vi "ReadIOIni.vi"(11 "IOPathIn":path) -> (3 "DIO":cluster{"DI=1":i32, "Name":string[]}[](array[cluster]))   [LabVIEW 2019]
uses:
  <vilib>/Utility/config.llb/Read Key (String).vi
  <vilib>/Utility/config.llb/NI_LVConfig.lvlib
panel:
  out "Numeric":i32
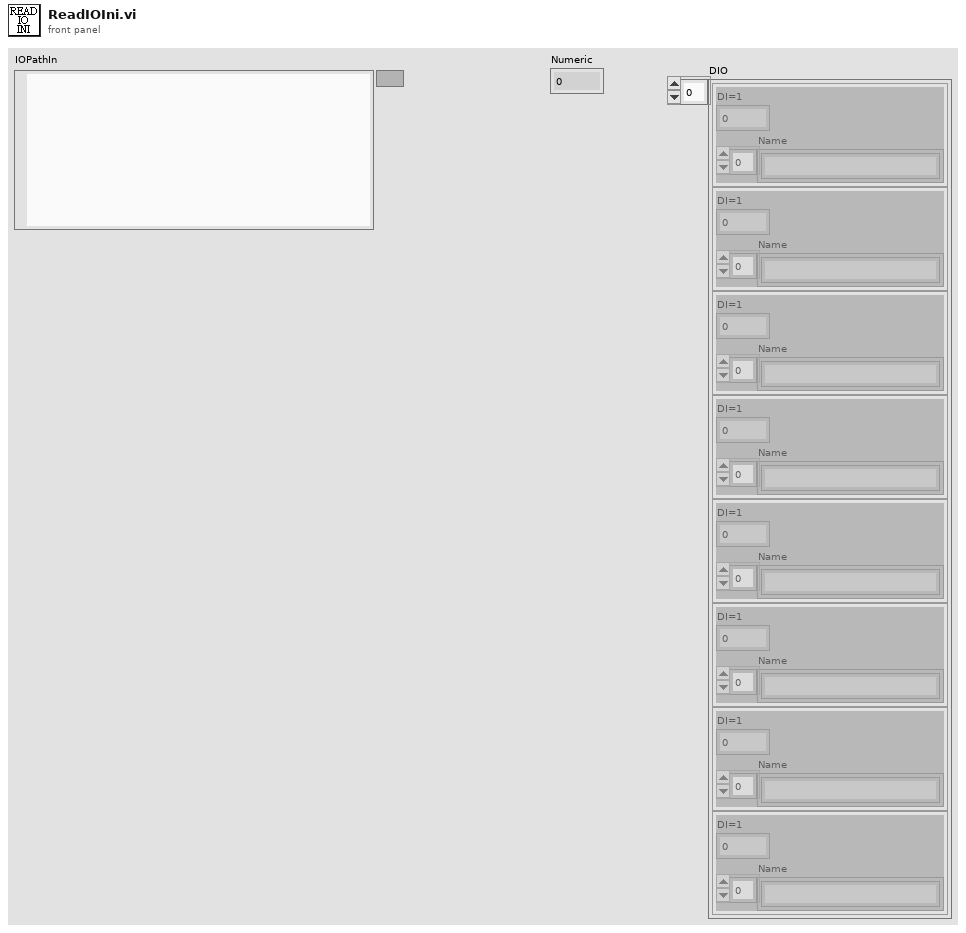
[diagram p1: front panel]
types:
  T1 = typedef "NI_LVConfig.lvlib/Config Data RefNum.ctl" = refnum<k1>
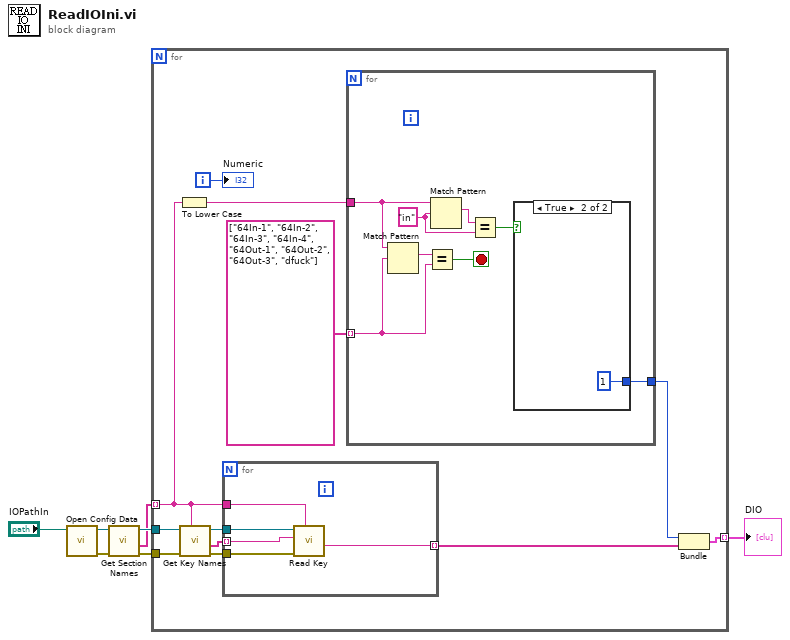
[diagram p0: block diagram]
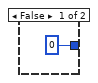
[diagram p2: hidden frame]
diagram:
  n1 = call <vilib>:"Open Config Data.vi"("configuration file path"="IOPathIn") -> ("error out"=w4:errorcluster, "refnum"=w7:T1)  [unwired: 8 in, 1 out]
  n2 = call <vilib>:"Get Section Names.vi"("error in (no error)"=w4, "refnum"=w7) -> ("error out"=w3:errorcluster, "section names"=w5:string[], "refnum out"=w6:T1)  [unwired: 7 in]
  n3 = for {
    tunnel: w6 -> [w19]
    tunnel: w5 -> [w12] mode=indexing
    tunnel: w3 -> [w16]
    tunnel: [w10] -> w1 mode=indexing
    i -> [w14]
    n4 = To Lower Case(string=w12) -> (all lower case string=w9:string)
    n5 = call <vilib>:"Get Key Names.vi"("section"=w12, "error in (no error)"=w16, "refnum"=w19) -> ("error out"=w15:errorcluster, "key names"=w18:string[], "refnum out"=w17:T1)  [unwired: 5 in, 1 out]
    n6 = for {
      tunnel: w12 -> [w34]
      tunnel: w18 -> [w33] mode=indexing
      tunnel: w17 -> [w32]
      tunnel: w15 -> [w31]
      tunnel: [w30] -> w11 mode=indexing
      n7 = call-poly <vilib>:"Read Key.vi"("section"=w34, "error in (no error)"=w31, "key"=w33, "refnum"=w32) -> ("value"=w30:string)  [unwired: 4 in, 3 out]
    }
    n8 = for {
      tunnel: string[] ["64In-1", "64In-2", "64In-3", "64In-4", "64Out-1", "64Out-2", "64Out-3", "dfuck"] -> [w26] mode=indexing
      tunnel: w9 -> [w24]
      tunnel: [w20] -> w8
      stop <- w25 stop-if-true
      w22 = "in" ("regular expression")
      n9 = Match Pattern(string=w24, regular expression=w26) -> (match substring=w27:string)  [unwired: 1 in, 3 out]
      n10 = Equal?(x=w27, y=w26) -> (x = y?=w25:bool)
      n11 = Match Pattern(string=w24, regular expression=w22) -> (match substring=w23:string)  [unwired: 1 in, 3 out]
      n12 = Equal?(x=w23, y=w22) -> (x = y?=w21:bool)
      n13 = case shown="True" w21 {
        tunnel: [0 1] -> w20
        frame False {
        }
        frame True {
        }
      }
    }
    n14 = Bundle(w8, w11) -> (w10:cluster{i32, string[]})  [unwired: 1 in]
    "Numeric" <- w14
  }
  "DIO" <- w1
